vi "CohortInitialize.vi"(10 "Pulse Configuration":T1={"Charge Balance"=TRUE, "Signal Amplitude"=5, "Signal Frequency [Hz]"=10, "Signal Duration [s]"=1.0, "Delay Time [s]"=0.0, "Pulse Width [s]"=0.005} {"Pulse Width [s]" format="%0.2p"; "Delay Time [s]" format="%0.2p"; "Signal Amplitude" format="%0.0p"; "Signal Duration [s]" format="%0.2p"}) -> (0 "error out":errorcluster, 3 "Cohort out":refnum<class "Cohort.lvclass">)   [LabVIEW 2012, in "Cohort.lvclass"]
uses:
  Cohort.lvclass
  Electrode.lvclass
  PulseConfig.ctl
  StimulCtrls.lvlib
panel:
  in  "error in (no error)":errorcluster
  in  "Cohort in":refnum<class "Cohort.lvclass">
  in  "Electrode #":u8=16
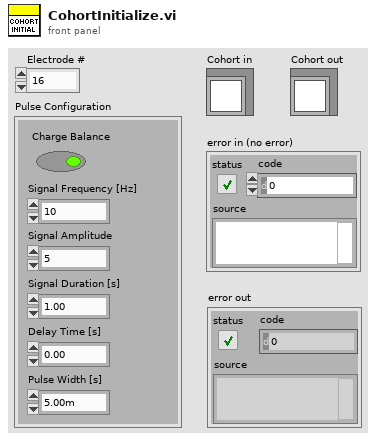
[diagram p1: front panel]
types:
  T1 = typedef "StimulCtrls.lvlib/PulseConfig.ctl" = cluster{"Charge Balance":bool, "Signal Amplitude":u32, "Signal Frequency [Hz]":u8, "Signal Duration [s]":sgl, "Delay Time [s]":sgl, "Pulse Width [s]":sgl}
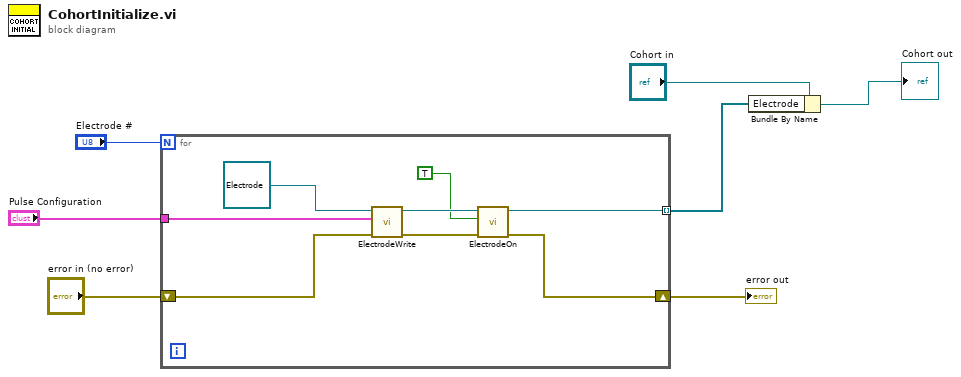
[diagram p0: block diagram]
diagram:
  n1 = for {
    N: "Electrode #" -> [_]
    tunnel: "Pulse Configuration" -> [w14]
    shift-right: [w11] -> w5
    shift-left: "error in (no error)" -> [w13]
    tunnel: [w8] -> w3 mode=indexing
    n2 = call "ElectrodeWrite.vi"("error in (no error)"=w13, "Pulse Configuration"=w14, "Electrode in"=refnum<class "Electrode.lvclass"> refnum ("Electrode.lvclass")) -> ("error out"=w12:errorcluster, "Electrode out"=w10:refnum<class "Electrode.lvclass">)  [unwired: 7 in]
    n3 = call-dynamic "ElectrodeOn.vi"("error in (no error)"=w12, "Electrode On"=TRUE, "Electrode in"=w10) -> ("error out"=w11:errorcluster, "Electrode out"=w8:refnum<class "Electrode.lvclass">)  [unwired: 7 in]
  }
  "error out" <- w5
  n4 = Bundle By Name(cluster="Cohort in", "Electrode"=w3) -> (→"Cohort out":refnum<class "Cohort.lvclass">)
